vi "BatchWrite.vi"(5 "输入数组":i16[](array[numeric])=[1234, 12592, 0, 19328, 0, 0, 27380, 824, 28836, 16709] format="%04x", 7 "软元件":string="D0", 8 "错误输入":errorcluster caption="错误输入（无错误）", 11 "连接输入":T1) -> (0 "错误输出":errorcluster, 1 "错误代码":u16, 2 "写入状态":bool, 3 "连接ID OUT":refnum<k16>)   [LabVIEW 2018]
panel:
  out "发送字符串":string
  out "数据输出":string
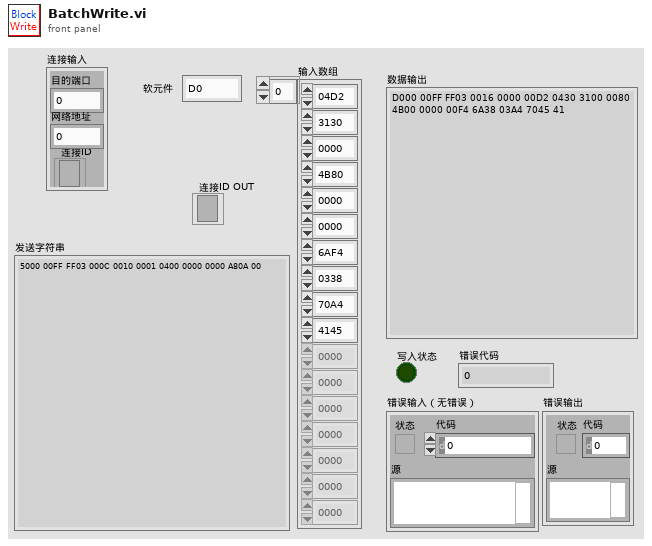
[diagram p1: front panel]
types:
  T1 = cluster{"目的端口":u16, "网络地址":u32, "连接ID":refnum<k16>}
  T2 = enum16{"big-endian, network order", "native, host order", "little-endian"}
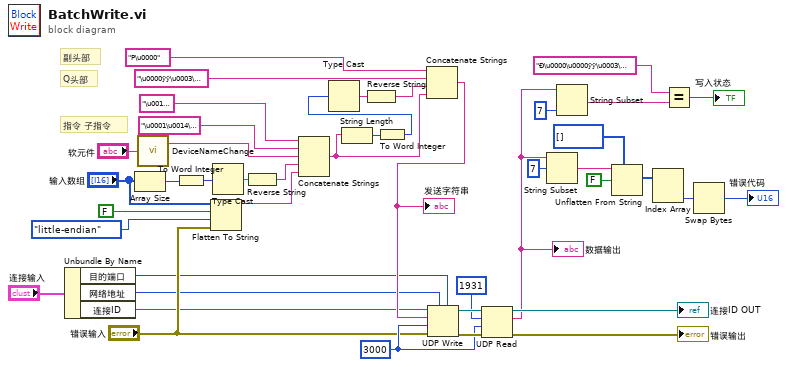
[diagram p0: block diagram]
diagram:
  w38 = 3000 ("超时毫秒(25000)")
  # "指令 子指令"
  # "Q头部"
  # "副头部"
  n1 = Unbundle By Name("连接输入") -> ("目的端口"=w4:u16, "网络地址"=w3:u32, "连接ID"=w2:refnum<k16>)
  n2 = Array Size(array="输入数组") -> (size(s)=w17:i32)
  n3 = call "DeviceNameChange.vi"("软元件"="软元件") -> ("字符串"=w29:string)  [unwired: 1 out]
  n4 = To Word Integer(number=w17) -> (16bit integer=w18:i16)
  n5 = Flatten To String(anything="输入数组", prepend array or string size? (T)=FALSE ("预置数组或字符串大小？ (T)"), byte order (0:big-endian, network order)=T2."little-endian" ("字节顺序(0:big-endian, network order)"), error in (no error)="错误输入") -> (data string=w25:string)  [unwired: 2 out]
  n6 = Type Cast(x=w18) -> (*(type *) &x=w43:string)  [unwired: 1 in]
  n7 = Reverse String(1:w43) -> (0:w42:string)
  n8 = Concatenate Strings("\u0010\u0000", "\u0001\u0014\u0000\u0000", w29, w42, w25) -> (w24:string)
  n9 = String Length(string=w24) -> (length=w20:i32)
  n10 = To Word Integer(number=w20) -> (16bit integer=w19:i16)
  n11 = Type Cast(x=w19) -> (*(type *) &x=w21:string)  [unwired: 1 in]
  n12 = Reverse String(1:w21) -> (0:w22:string)
  n13 = Concatenate Strings("P\u0000", "\u0000ÿÿ\u0003\u0000", w22, w24) -> (w23:string)
  "发送字符串" <- w23
  n14 = UDP Write(address=w3, port or service name=w4, connection ID=w2, data in=w23, 8:"错误输入", 9:w38) -> (error out=w39:errorcluster, 3:w40:refnum<k16>)
  n15 = UDP Read(connection ID=w40, max size (548)=1931 ("最大值(548)"), timeout ms (25000)=w38, 8:w39) -> (data out=w13:string, error out=→"错误输出":errorcluster, 3:→"连接ID OUT":refnum<k16>)  [unwired: 2 out]
  "数据输出" <- w13
  n16 = String Subset(string=w13, offset (0)=7 ("偏移量(0)")) -> (substring=w10:string)  [unwired: 1 in]
  n17 = String Subset(string=w13, length (rest)=7 ("长度（剩余）")) -> (substring=w34:string)  [unwired: 1 in]
  n18 = Unflatten From String(type=u16[] [], binary string=w10, data includes array or string size? (T)=FALSE ("数据中包含数组或字符串大小？(T)")) -> (value=w9:u16[])  [unwired: 2 in, 2 out]
  n19 = Index Array(array=w9) -> (element #2=w8:u16)  [unwired: 2 in, 1 out]
  n20 = Equal?(x="Ð\u0000\u0000ÿÿ\u0003\u0000", y=w34) -> (x = y?=→"写入状态":bool)
  n21 = Swap Bytes(anything=w8) -> (byte swapped=→"错误代码":u16)
